vi "Check Info.vi"(0 "VISA Resource Name":refnum<visa-resource-name>, 5 "Information Type (4:OPTION)":T1(ring)=enum."OPTION", 11 "error in (no error)":errorcluster {"code" format="%.0x"}) -> (4 "VISA Resource Name Out":refnum<visa-resource-name>, 6 "Information":string, 15 "error out":errorcluster {"code" format="%.0x"})   [LabVIEW 2012, in "Agilent ESG Series.lvlib"]
doc: "This VI is used query the instrument about various operational and tracking data."
uses:
  <instrlib>/Agilent ESG Series/Agilent ESG Series.lvlib
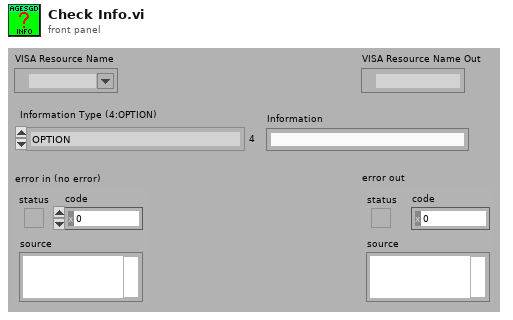
[diagram p1: front panel]
types:
  T1 = enum16{"ATTENUATOR CYCLE", "DISPLAY TIME-ON", "POWER CYCLE", "REVERSE POWER PROTECTION TRIPS", "OPTION", "SERIAL NUMBER AND FIRMWARE", "INSTRUMENT TIME-ON"}
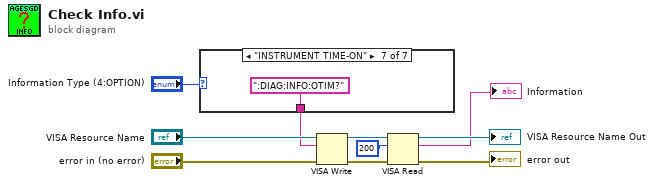
[diagram p0: block diagram]
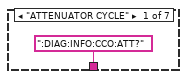
[diagram p2: hidden frame]
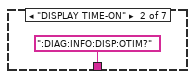
[diagram p3: hidden frame]
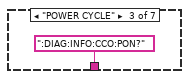
[diagram p4: hidden frame]
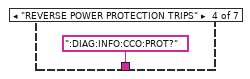
[diagram p5: hidden frame]
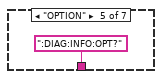
[diagram p6: hidden frame]
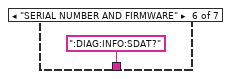
[diagram p7: hidden frame]
diagram:
  n1 = case shown="\"INSTRUMENT TIME-ON\"" "Information Type (4:OPTION)" {
    tunnel: [":DIAG:INFO:CCO:ATT?" ":DIAG:INFO:DISP:OTIM?" ":DIAG:INFO:CCO:PON?" ":DIAG:INFO:CCO:PROT?" ":DIAG:INFO:OPT?" ":DIAG:INFO:SDAT?" ":DIAG:INFO:OTIM?"] -> w8
    frame "ATTENUATOR CYCLE" {
    }
    frame "DISPLAY TIME-ON" {
    }
    frame "POWER CYCLE" {
    }
    frame "REVERSE POWER PROTECTION TRIPS" {
    }
    frame "OPTION" {
    }
    frame "SERIAL NUMBER AND FIRMWARE" {
    }
    frame "INSTRUMENT TIME-ON" {
    }
  }
  n2 = VISA Write(VISA resource name="VISA Resource Name", write buffer=w8, error in (no error)="error in (no error)") -> (VISA resource name out=w6:refnum<visa-resource-name>, error out=w5:errorcluster)  [unwired: 1 out]
  n3 = VISA Read(VISA resource name=w6, byte count=u32 200 ("byte count (0)"), error in (no error)=w5) -> (VISA resource name out=→"VISA Resource Name Out":refnum<visa-resource-name>, read buffer=→"Information":string, error out=→"error out":errorcluster)  [unwired: 1 out]
